vi "pco.camera_Live_ConvertSetting_Examples.vi"() -> ()   [LabVIEW 2019]
doc: "A short program to demonstrate the fundamentals of control and image acquision with the pco.camera series. The program records a sequence of images, with \"live\" updating, until the \"StopRecording\" button is pressed. Use ctrl-H for more help on the individual controls and indicators.\n\nCopyright 2004, 2010 The Cooke Corporation."
uses:
  pco.camera/Camera.lvclass
  pco.sdk/TimingControl/TimingControl.lvlib
  <vilib>/picture/picture.llb/Draw True-Color Pixmap.vi
  <vilib>/picture/picture.llb/Draw 8-Bit Pixmap.vi
panel:
  out "colormap(U8)":u32[](array[numeric])
  out "Image(U16)":u16[][](graph)
  in  "Zoom [%]":i32(c297)=26
  out "Image":picture
  in  "settingsChanged":bool
  in  "Trigger":bool
  in  "LUT File":path
  in  "data_format":T1(ring)=enum."RGBA8"
  in  "Auto Range":bool
  out "rawImage":u16[][](array[numeric])
  in  "iContrast [%]":i32 min=-100 max=99 step=1
  in  "Gamma":dbl=1.0 min=0.01 max=10.0 step=0.01 format="%.2f"
  in  "whiteBalance":bool
  in  "iScale_max":u16=60000 step=1
  in  "iScale_min":u16=200 step=1
  in  "Image Index":u32 max=9
  out "Recorded Images":u32
  in  "TriggerMode":T2(ring)
  in  "Quit":bool
  out "Error":errorcluster {"code" format="%x"}
  in  "Stop Record":bool
  out "Recording On":bool
  in  "roiY1":u64=2 min=1 max=2160 step=1
  in  "roiX1":u64=2 min=1 max=2560 step=1
  in  "roiY0":u64=1 min=1 max=2159 step=1
  in  "roiX0":u64=1 min=1 max=2559 step=1
  out "Image Height":u64
  out "Image Width":u64
  in  "dwImgCount":u32=10 caption="Required Number of Images" max=2397
  in  "Exposure Time [s]":dbl=0.010000000000000002 min=0.0005 max=2.0 step=0.001
  # "This example demonstrates the image acquisition with one camera in ring buffer mode together with a live display of the latest images during record. After record is stopped, the images can be addressed by index.\nAdditionally the image convert settings can be adjusted at any time\nNote that this example will not be fail save, i.e. doesnt react on errors, just handles them forward to the end\n\nUsage:\nSelect your required image count and the camera setup before you start the program.\nOnce started, the camera class will be initialized and images will be recorded and displayed automatically\nYou can stop the images by pressing stop record.\nAfter stopped, the image at the selected index will be read out\nTo finish the program click on quit application, this will force an exit of the camera class\nYou can change your required ROI after and also during the record."
  # "pco.labview"
  # "Camera Setup"
  # "Recording Control"
  # "Parameters for image readout"
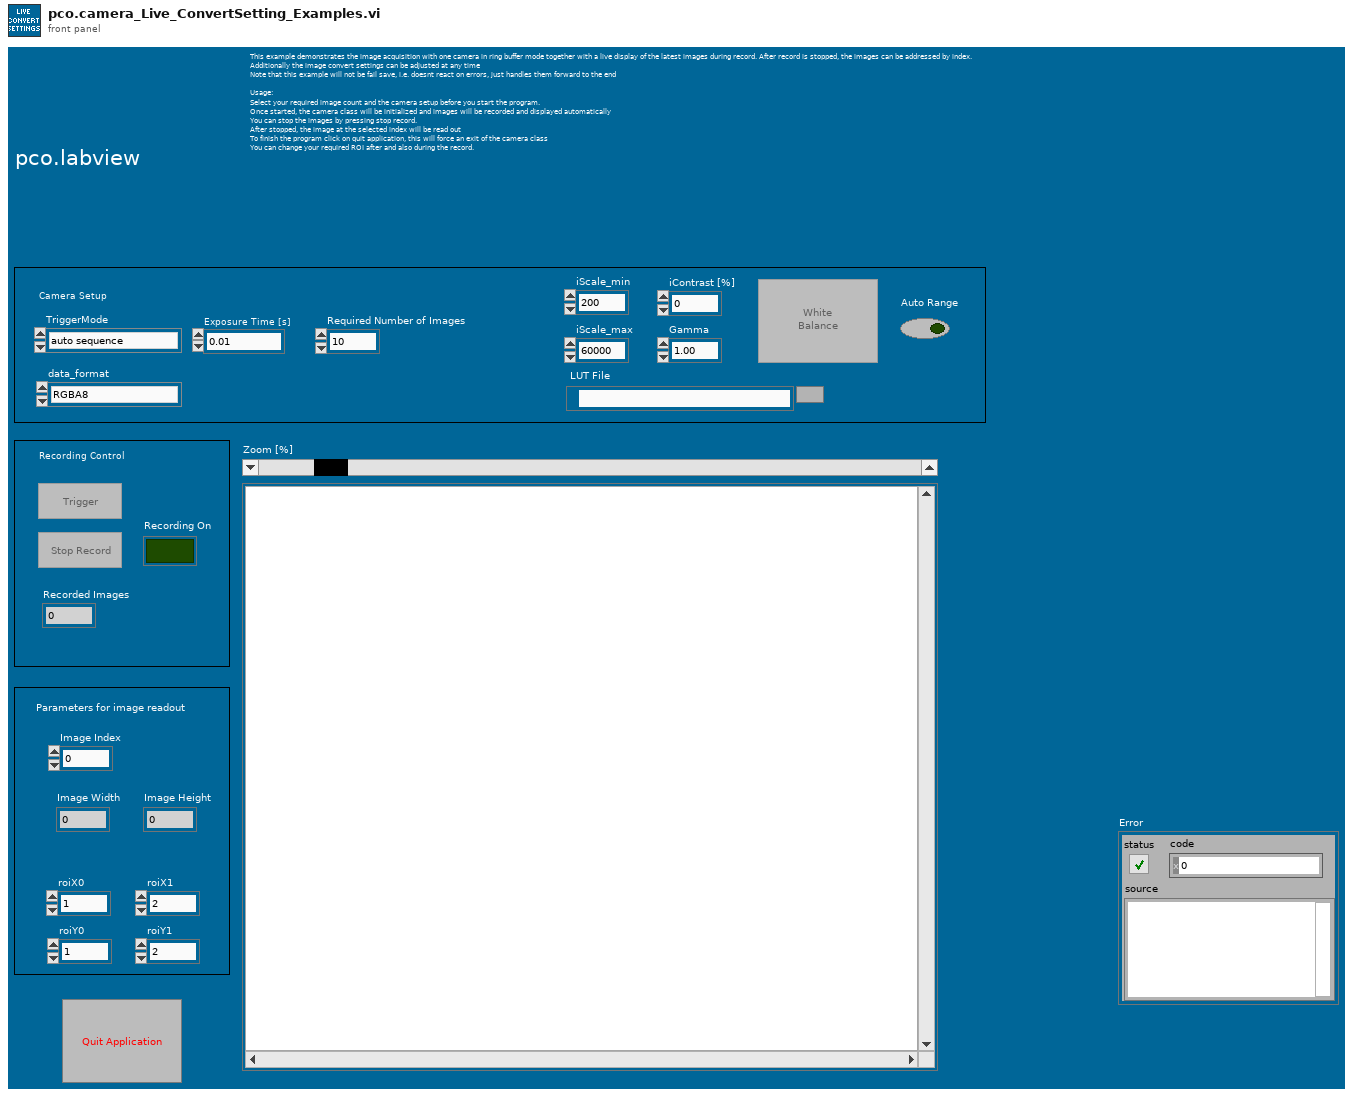
[diagram p1: front panel]
types:
  T1 = enum16{"Undefined", "Mono8", "Mono16", "BGRA8", "RGBA8", "BGRA16", "RGBA16", "CompressedMono8"}
  T2 = enum16{"auto sequence", "software trigger", "external exposure start", "external exposure control"}
  T3 = enum16{"sequence", "sequence non blocking", "ring buffer", "fifo", "sequence_dpcore", "sequence_non_blocking_dpcore", "ring_buffer_dpcore", "fifo_dpcore", "tif", "multitif", "pcoraw", "b16", "dicom", "multidicom"}
  T4 = enum8{"Enabled", "Disabled", "Disabled and Grayed Out"}
  T5 = cluster{"serial":u32, "type":u16, "sub_type":u16, "interface_type":u16, "bit_resolution":u16, "min_exposure_time_s":dbl, "max_exposure_time_s":dbl, "min_exposure_step_s":dbl, "min_delay_time_s":dbl, "max_delay_time_s":dbl, "min_delay_step_s":dbl, "min_width":u64, "min_height":u64, "max_width":u64, "max_height":u64, "roi_step_horz":u64, "roi_step_vert":u64, "roi_symmetric_horz":bool, "roi_symmetric_vert":bool, "has_timestamp_mode":bool, "has_timestamp_mode_ascii_only":bool, "pixelrate_vec":u32[], "has_acquire_mode":bool, "has_ext_acquire_mode":bool, "has_metadata_mode":bool, "has_ram":bool, "binning_horz_vec":u16[], "binning_vert_vec":u16[]}
  T6 = typedef "Camera.lvclass/binning.ctl" = cluster{"vert":u16, "horz":u16}
  T7 = cluster{"exposure_time_s":dbl, "delay_time_s":dbl, "roi":cluster{"x0":u64, "y0":u64, "x1":u64, "y1":u64}, "timestamp_mode":u16, "pixelrate":u32, "trigger_mode":u16, "acquire_mode":u16, "metadata_mode":u16, "noisefilter_mode":u16, "binning":T6}
  T8 = cluster{"sharpen":bool, "adaptive_sharpen":bool, "flip_vertical":bool, "auto_minmax":bool, "min_limit":u16, "max_limit":u16, "gamma":dbl, "contrast":i32, "pco_debayer_algorithm":bool, "color_temperature":i32, "color_saturation":i32, "color_vibrance":i32, "color_tint":i32, "lut_file":path}
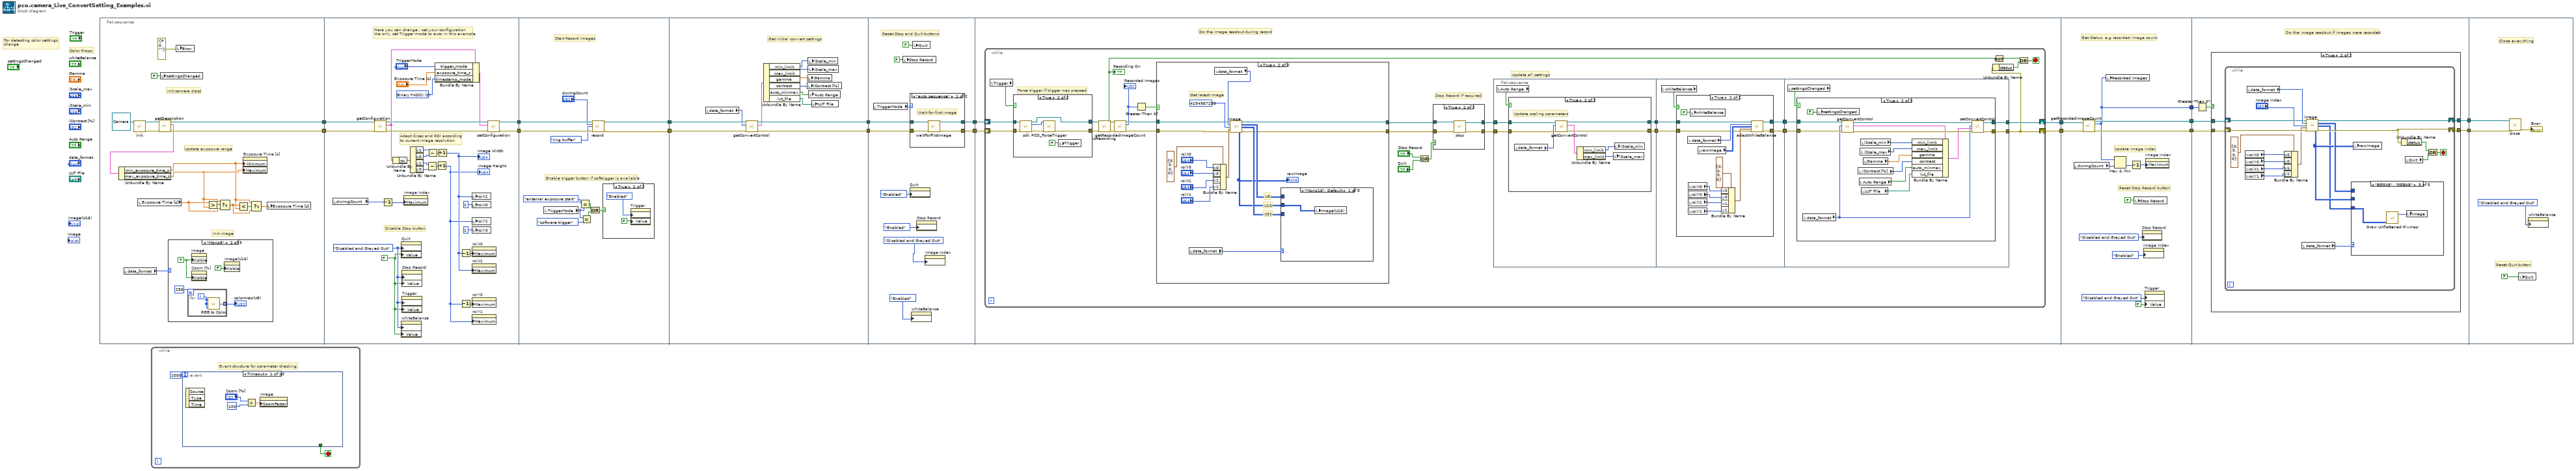
[diagram p0: block diagram]
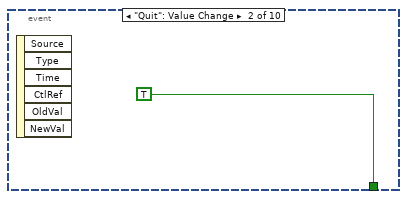
[diagram p2: hidden frame]
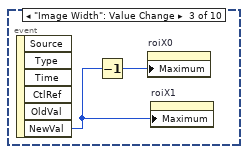
[diagram p3: hidden frame]
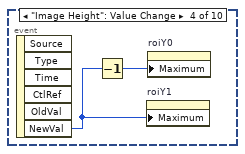
[diagram p4: hidden frame]
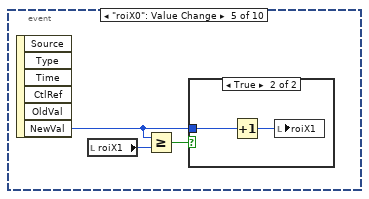
[diagram p5: hidden frame]
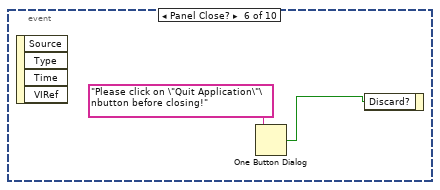
[diagram p7: hidden frame]
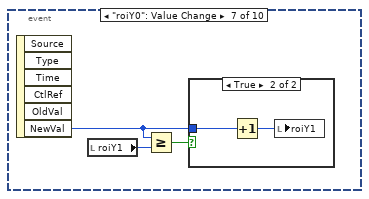
[diagram p8: hidden frame]
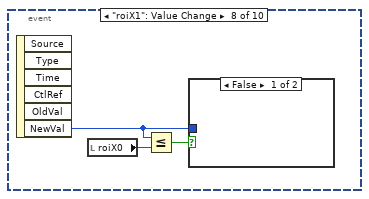
[diagram p10: hidden frame]
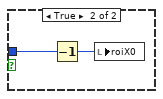
[diagram p11: hidden frame]
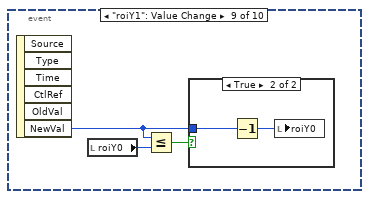
[diagram p12: hidden frame]
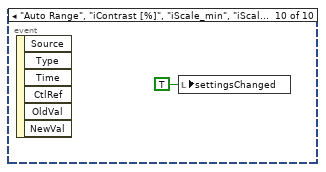
[diagram p14: hidden frame]
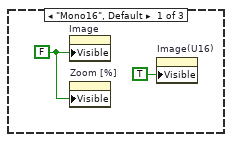
[diagram p15: hidden frame]
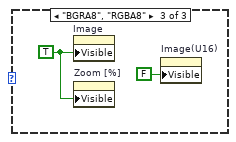
[diagram p16: hidden frame]
diagram:
  # "For detecting color settings\nchange"
  # "Color Props"
  n1 = flat-sequence {
    tunnel: [w24] -> w7
    tunnel: [w23] -> w6
    tunnel: [w48] -> w17
    tunnel: [w52] -> w16
    tunnel: w7 -> [w47]
    tunnel: w6 -> [w46]
    tunnel: w17 -> [w82]
    tunnel: w16 -> [w83]
    tunnel: [w79] -> w11
    tunnel: [w80] -> w8
    tunnel: w11 -> [w96]
    tunnel: [w91] -> w10
    tunnel: [w97] -> w9
    tunnel: w8 -> [w87]
    tunnel: w10 -> [w104]
    tunnel: w9 -> [w105]
    tunnel: [w103] -> w15
    tunnel: [w100] -> w2
    tunnel: w15 -> [w118]
    tunnel: [w117] -> w14
    tunnel: [w116] -> w5
    tunnel: w2 -> [w115]
    tunnel: w14 -> [w253]
    tunnel: [w251] -> w13
    tunnel: w5 -> [w246]
    tunnel: [w245] -> w4
    tunnel: [w244] -> w1
    tunnel: w13 -> [w262]
    tunnel: [w261] -> w12
    tunnel: w4 -> [w260]
    tunnel: [w259] -> w3
    tunnel: w1 -> [w257]
    tunnel: w12 -> [w297]
    tunnel: w3 -> [w294]
    frame #0 {
      # "Init image"
      # "Init camera class"
      # "Update exposure range"
      n2 = local read "data_format"() -> (w19:T1)
      n3 = call-dynamic "init.vi"("Camera in"=refnum<class "Camera.lvclass"> refnum) -> ("Camera out"=w25:refnum<class "Camera.lvclass">, "error out"=w26:errorcluster)  [unwired: 8 in]
      n4 = local read "Exposure Time [s]"() -> (w32:dbl)
      n5 = call-dynamic "getDescription.vi"("error in (no error)"=w26, "Camera in"=w25) -> ("error out"=w23:errorcluster, "description"=w22:T5, "Camera out"=w24:refnum<class "Camera.lvclass">)  [unwired: 7 in]
      n6 = Unbundle By Name(w22) -> ("min_exposure_time_s"=w21:dbl, "max_exposure_time_s"=w20:dbl)
      n7 = local write "settingsChanged"(FALSE ("settingsChanged")) -> ()
      n8 = case shown="\"Mono8\"" w19 {
        frame "Mono16", Default {
          w34 = FALSE ("Visible")
          n9 = property on="Image" class="Pict"("Visible"=w34) -> ()  [unwired: 2 in, 2 out]
          n10 = property on="Zoom [%]" class="Scroll (strict)"("Visible"=w34) -> ()  [unwired: 2 in, 2 out]
          n11 = property on="Image(U16)" class="IntGraph (strict)"("Visible"=TRUE) -> ()  [unwired: 2 in, 2 out]
        }
        frame "Mono8" {
          w36 = TRUE ("Visible")
          n12 = for {
            N: 256 -> [_]
            tunnel: [w40] -> w39 mode=indexing
            i -> [w41]
            n13 = call <vilib>:"RGB to Color.vi"("B"=w41, "G"=w41, "R"=w41) -> ("Color"=w40:u32)
          }
          "colormap(U8)" <- w39
          n14 = property on="Image" class="Pict"("Visible"=w36) -> ()  [unwired: 2 in, 2 out]
          n15 = property on="Zoom [%]" class="Scroll (strict)"("Visible"=w36) -> ()  [unwired: 2 in, 2 out]
          n16 = property on="Image(U16)" class="IntGraph (strict)"("Visible"=FALSE) -> ()  [unwired: 2 in, 2 out]
        }
        frame "BGRA8", "RGBA8" {
          w42 = TRUE ("Visible")
          n17 = property on="Image" class="Pict"("Visible"=w42) -> ()  [unwired: 2 in, 2 out]
          n18 = property on="Zoom [%]" class="Scroll (strict)"("Visible"=w42) -> ()  [unwired: 2 in, 2 out]
          n19 = property on="Image(U16)" class="IntGraph (strict)"("Visible"=FALSE) -> ()  [unwired: 2 in, 2 out]
        }
      }
      n20 = local write "Error"(errorcluster {"status"=FALSE, "code"=0, "source"=""} ("error IO")) -> ()
      n21 = Greater?(x=w32, y=w20) -> (0:w33:bool)
      n22 = Select(t=w20, s=w33, f=w32) -> (s? t:f=w30:dbl)
      n23 = Less?(x=w30, y=w21) -> (x < y?=w31:bool)
      n24 = property on="Exposure Time [s]" class="DigNum (strict)"("Minimum"=w21, "Maximum"=w20) -> ()  [unwired: 2 in, 2 out]
      n25 = Select(t=w21, s=w31, f=w30) -> (s? t:f=w29:dbl)
      n26 = local write "Exposure Time [s]"(w29) -> ()
    }
    frame #1 {
      w58 = u16 2 items=["OFF", "Binary", "Binary+ASCII", "ASCII"] ("wTimeStampMode")
      w44 = FALSE ("Stop")
      w45 = T4."Disabled and Grayed Out" ("Disabled")
      # "Disable Stop button"
      # "Adapt Sizes and ROI according\nto current image resolution"
      # "Here you can change / set your configuration\nWe only set Trigger mode to auto in this example"
      n27 = local read "dwImgCount"() -> (w59:u32)
      n28 = call-dynamic "getConfiguration.vi"("error in (no error)"=w46, "Camera in"=w47) -> ("error out"=w53:errorcluster, "configuration"=w64:T7, "Camera out"=w55:refnum<class "Camera.lvclass">)  [unwired: 7 in]
      n29 = Decrement(x=w59) -> (x-1=w49:u32)
      n30 = Unbundle By Name(w64) -> ("roi"=w65:cluster{"x0":u64, "y0":u64, "x1":u64, "y1":u64})
      n31 = property on="Quit" class="Bool (strict)"("DisabledEnum"=w45, "Value"=w44) -> ()  [unwired: 2 in, 2 out]
      n32 = property on="whiteBalance" class="Bool (strict)"("DisabledEnum"=w45, "Value"=w44) -> ()  [unwired: 2 in, 2 out]
      n33 = property on="Stop Record" class="Bool (strict)"("DisabledEnum"=w45, "Value"=w44) -> ()  [unwired: 2 in, 2 out]
      n34 = property on="Trigger" class="Bool (strict)"("DisabledEnum"=w45, "Value"=w44) -> ()  [unwired: 2 in, 2 out]
      n35 = property on="Image Index" class="DigNum (strict)"("Maximum"=w49) -> ()  [unwired: 2 in, 2 out]
      n36 = Unbundle By Name(w65) -> ("x1"=w67:u64, "x0"=w66:u64, "y1"=w69:u64, "y0"=w68:u64)
      n37 = Subtract(x=w69, y=w68) -> (x-y=w71:u64)
      n38 = Subtract(x=w67, y=w66) -> (x-y=w70:u64)
      n39 = Bundle By Name(cluster=w64, "trigger_mode"="TriggerMode", "exposure_time_s"="Exposure Time [s]", "timestamp_mode"=w58) -> (w54:T7)
      n40 = Increment(x=w71) -> (x+1=w50:u64)
      "Image Height" <- w50
      n41 = Increment(x=w70) -> (x+1=w51:u64)
      "Image Width" <- w51
      n42 = Decrement(x=w51) -> (x-1=w62:u64)
      n43 = Decrement(x=w50) -> (x-1=w63:u64)
      n44 = local write "roiX1"(w51) -> ()
      n45 = local write "roiX0"(u64 1 ("roiY0")) -> ()
      n46 = local write "roiY1"(w50) -> ()
      n47 = local write "roiY0"(u64 1 ("roiY0")) -> ()
      n48 = property on="roiX0" class="DigNum (strict)"("Maximum"=w62) -> ()  [unwired: 2 in, 2 out]
      n49 = property on="roiX1" class="DigNum (strict)"("Maximum"=w51) -> ()  [unwired: 2 in, 2 out]
      n50 = property on="roiY0" class="DigNum (strict)"("Maximum"=w63) -> ()  [unwired: 2 in, 2 out]
      n51 = property on="roiY1" class="DigNum (strict)"("Maximum"=w50) -> ()  [unwired: 2 in, 2 out]
      n52 = call-dynamic "setConfiguration.vi"("error in (no error)"=w53, "configuration"=w54, "Camera in"=w55) -> ("error out"=w52:errorcluster, "Camera out"=w48:refnum<class "Camera.lvclass">)  [unwired: 7 in]
    }
    frame #2 {
      # "Enable trigger button if softtrigger is available"
      # "Start Record Images"
      n53 = local read "TriggerMode"() -> (w77:T2)
      n54 = Equal?(x=T2."external exposure start" ("TriggerMode"), y=w77) -> (x = y?=w74:bool)
      n55 = Equal?(x=w77, y=T2."software trigger" ("TriggerMode")) -> (x = y?=w73:bool)
      n56 = Or(x=w74, y=w73) -> (x .or. y?=w75:bool)
      n57 = call-dynamic "record.vi"("Camera in"=w82, "num_images"="dwImgCount", "record_mode"=T3."ring buffer", "error in (no error)"=w83) -> ("Camera out"=w80:refnum<class "Camera.lvclass">, "error out"=w79:errorcluster)  [unwired: 10 in]
      n58 = case shown="True" w75 {
        frame False {
        }
        frame True {
          n59 = property on="Trigger" class="Bool (strict)"("DisabledEnum"=T4."Enabled" ("Disabled"), "Value"=FALSE ("Trigger")) -> ()  [unwired: 2 in, 2 out]
        }
      }
    }
    frame #3 {
      # "Get initial convert settings"
      n60 = local read "data_format"() -> (w86:T1)
      n61 = call-dynamic "getConvertControl.vi"("error in (no error)"=w96, "data_format"=w86, "Camera in"=w87) -> ("error out"=w91:errorcluster, "convert_control"=w95:T8, "Camera out"=w97:refnum<class "Camera.lvclass">)  [unwired: 6 in]
      n62 = Unbundle By Name(w95) -> ("min_limit"=w93:u16, "max_limit"=w92:u16, "gamma"=w94:dbl, "contrast"=w90:i32, "auto_minmax"=w89:bool, "lut_file"=w88:path)
      n63 = local write "iContrast [%]"(w90) -> ()
      n64 = local write "Gamma"(w94) -> ()
      n65 = local write "iScale_min"(w93) -> ()
      n66 = local write "iScale_max"(w92) -> ()
      n67 = local write "Auto Range"(w89) -> ()
      n68 = local write "LUT File"(w88) -> ()
    }
    frame #4 {
      # "Reset Stop and Quit buttons"
      n69 = local read "TriggerMode"() -> (w98:T2)
      n70 = local write "Stop Record"(FALSE ("Stop Record")) -> ()
      n71 = case shown="\"auto sequence\"" w98 {
        tunnel: w105 -> [w112 w114]
        tunnel: w104 -> [w111 w113]
        tunnel: [w110 w113] -> w103
        tunnel: [w109 w114] -> w100
        frame "auto sequence" {
          # "Wait for first image"
          n72 = call-dynamic "waitForFirstImage.vi"("error in (no error)"=w111, "Camera in"=w112) -> ("error out"=w110:errorcluster, "Camera out"=w109:refnum<class "Camera.lvclass">)  [unwired: 8 in]
        }
        frame Default {
          # "Don't wait \nif we trigger"
        }
      }
      n73 = property on="Quit" class="Bool (strict)"("DisabledEnum"=T4."Enabled" ("Disabled")) -> ()  [unwired: 2 in, 2 out]
      n74 = property on="whiteBalance" class="Bool (strict)"("DisabledEnum"=T4."Enabled" ("Disabled")) -> ()  [unwired: 2 in, 2 out]
      n75 = local write "Quit"(FALSE ("Stop")) -> ()
      n76 = property on="Stop Record" class="Bool (strict)"("DisabledEnum"=T4."Enabled" ("Disabled")) -> ()  [unwired: 2 in, 2 out]
      n77 = property on="Image Index" class="DigNum (strict)"("DisabledEnum"=T4."Disabled and Grayed Out" ("Disabled")) -> ()  [unwired: 2 in, 2 out]
    }
    frame #5 {
      # "Do the image readout during record"
      n78 = while {
        shift-right: [w128] -> w117
        shift-left: w118 -> [w131]
        shift-right: [w134] -> w116
        shift-left: w115 -> [w132]
        stop <- w146 stop-if-true
        # "Stop Record if required"
        # "Force trigger if trigger was pressed"
        # "Update all settings"
        n79 = local read "Trigger"() -> (w133:bool)
        n80 = case shown="True" w133 {
          tunnel: w132 -> [w178 w183]
          tunnel: w131 -> [w177 w182]
          tunnel: [w178 w181] -> w130
          tunnel: [w177 w180] -> w129
          frame False {
          }
          frame True {
            n81 = call-dynamic "sdk.vi"("Camera in"=w183, "error in (no error)"=w182) -> ("Camera out"=w181:refnum<class "Camera.lvclass">, "sdk"=w184:u64, "error out"=w185:errorcluster)  [unwired: 11 in]
            n82 = call "PCO_ForceTrigger.vi"("error in (no error)"=w185, "ph"=w184) -> ("error out"=w180:errorcluster)  [unwired: 6 in, 3 out]
            n83 = local write "Trigger"(FALSE ("Trigger")) -> ()
          }
        }
        n84 = call-dynamic "isRecording.vi"("Camera in"=w130, "error in (no error)"=w129) -> ("Camera out"=w142:refnum<class "Camera.lvclass">, "recording"=w144:bool, "error out"=w141:errorcluster)  [unwired: 11 in]
        "Recording On" <- w144
        n85 = call-dynamic "getRecordedImageCount.vi"("Camera in"=w142, "error in (no error)"=w141) -> ("Camera out"=w139:refnum<class "Camera.lvclass">, "recorded_image_count"=w127:u32, "error out"=w140:errorcluster)  [unwired: 11 in]
        "Recorded Images" <- w127
        n86 = Greater Than 0?(x=w127) -> (x > 0?=w126:bool)
        n87 = case shown="True" w126 {
          tunnel: w140 -> [w153 w163]
          tunnel: w139 -> [w154 w157]
          tunnel: [w153 w155] -> w122
          tunnel: [w154 w156] -> w121
          frame False {
          }
          frame True {
            # "U32"
            # "U8"
            # "U16"
            # "Get latest image"
            n88 = local read "data_format"() -> (w158:T1)
            n89 = Bundle By Name(cluster=cluster{"x0":u64, "y0":u64, "x1":u64, "y1":u64} {"x0"=0, "y0"=0, "x1"=0, "y1"=0} ("roi"), "x0"="roiX0", "y0"="roiY0", "x1"="roiX1", "y1"="roiY1") -> (w166:cluster{"x0":u64, "y0":u64, "x1":u64, "y1":u64})
            n90 = local read "data_format"() -> (w162:T1)
            n91 = call-dynamic "image.vi"("Camera in"=w157, "data_format"=w162, "image_index"=u32 4294967295 ("dwImgIdx"), "roi"=w166, "error in (no error)"=w163) -> ("Camera out"=w156:refnum<class "Camera.lvclass">, "image (U8)"=w160:u8[][], "image (U32)"=w161:u32[][], "raw_image (U16)"=w159:u16[][], "error out"=w155:errorcluster)  [unwired: 3 in, 3 out]
            "rawImage" <- w159
            n92 = case shown="\"Mono16\", Default" w158 {
              tunnel: w161 -> [_ _ w176]
              tunnel: w160 -> [_ w173 _]
              tunnel: w159 -> [w171 _ _]
              frame "Mono16", Default {
                n93 = local write "Image(U16)"(w171) -> ()
              }
              frame "Mono8" {
                n94 = local read "colormap(U8)"() -> (w172:u32[])
                n95 = call-poly <vilib>:"Draw Unflattened Pixmap.vi"("data"=w173, "color table"=w172) -> ("new picture"=w174:picture)  [unwired: 7 in]
                n96 = local write "Image"(w174) -> ()
              }
              frame "BGRA8", "RGBA8" {
                n97 = call-poly <vilib>:"Draw Unflattened Pixmap.vi"("data (RGB format)"=w176) -> ("new picture"=w175:picture)  [unwired: 8 in]
                n98 = local write "Image"(w175) -> ()
              }
            }
          }
        }
        n99 = Or(x="Stop Record", y="Quit") -> (x .or. y?=w125:bool)
        n100 = case shown="True" w125 {
          tunnel: w122 -> [w148 w149]
          tunnel: [w147 w151] -> w120
          tunnel: [w148 w152] -> w119
          tunnel: w121 -> [w147 w150]
          frame False {
          }
          frame True {
            n101 = call-dynamic "stop.vi"("error in (no error)"=w149, "Camera in"=w150) -> ("error out"=w152:errorcluster, "Camera out"=w151:refnum<class "Camera.lvclass">)  [unwired: 8 in]
          }
        }
        n102 = flat-sequence {
          tunnel: w119 -> [w188]
          tunnel: w120 -> [w189]
          tunnel: [w187] -> w138
          tunnel: [w186] -> w137
          tunnel: w138 -> [w204]
          tunnel: w137 -> [w203]
          tunnel: [w202] -> w136
          tunnel: [w201] -> w135
          tunnel: w136 -> [w223]
          tunnel: w135 -> [w224]
          tunnel: [w222] -> w128
          tunnel: [w221] -> w134
          frame #0 {
            n103 = local read "Auto Range"() -> (w190:bool)
            n104 = case shown="True" w190 {
              tunnel: w189 -> [w192 w196]
              tunnel: w188 -> [w191 w195]
              tunnel: [w191 w194] -> w187
              tunnel: [w192 w193] -> w186
              frame False {
              }
              frame True {
                # "Update scaling parameters"
                n105 = local read "data_format"() -> (w200:T1)
                n106 = call-dynamic "getConvertControl.vi"("error in (no error)"=w195, "data_format"=w200, "Camera in"=w196) -> ("error out"=w194:errorcluster, "convert_control"=w197:T8, "Camera out"=w193:refnum<class "Camera.lvclass">)  [unwired: 6 in]
                n107 = Unbundle By Name(w197) -> ("min_limit"=w198:u16, "max_limit"=w199:u16)
                n108 = local write "iScale_max"(w199) -> ()
                n109 = local write "iScale_min"(w198) -> ()
              }
            }
          }
          frame #1 {
            n110 = local read "whiteBalance"() -> (w205:bool)
            n111 = case shown="True" w205 {
              tunnel: w204 -> [w206 w212]
              tunnel: w203 -> [w207 w211]
              tunnel: [w206 w210] -> w202
              tunnel: [w207 w209] -> w201
              frame False {
              }
              frame True {
                n112 = local read "data_format"() -> (w219:T1)
                n113 = local read "roiX0"() -> (w217:u64)
                n114 = local read "roiY0"() -> (w216:u64)
                n115 = local read "roiX1"() -> (w215:u64)
                n116 = local read "roiY1"() -> (w208:u64)
                n117 = local write "whiteBalance"(FALSE ("whiteBalance")) -> ()
                n118 = local read "rawImage"() -> (w218:u16[][])
                n119 = Bundle By Name(cluster=cluster{"x0":u64, "y0":u64, "x1":u64, "y1":u64} {"x0"=0, "y0"=0, "x1"=0, "y1"=0} ("roi"), "x0"=w217, "y0"=w216, "x1"=w215, "y1"=w208) -> (w214:cluster{"x0":u64, "y0":u64, "x1":u64, "y1":u64})
                n120 = call-dynamic "adaptWhiteBalance.vi"("Camera in"=w211, "data_format"=w219, "raw_image (U16)"=w218, "roi"=w214, "error in (no error)"=w212) -> ("Camera out"=w209:refnum<class "Camera.lvclass">, "error out"=w210:errorcluster)  [unwired: 9 in]
              }
            }
          }
          frame #2 {
            n121 = local read "settingsChanged"() -> (w225:bool)
            n122 = case shown="True" w225 {
              tunnel: w224 -> [w227 w233]
              tunnel: w223 -> [w226 w232]
              tunnel: [w226 w229] -> w222
              tunnel: [w227 w228] -> w221
              frame False {
              }
              frame True {
                n123 = local read "data_format"() -> (w231:T1)
                n124 = local write "settingsChanged"(FALSE ("whiteBalance")) -> ()
                n125 = call-dynamic "getConvertControl.vi"("error in (no error)"=w232, "data_format"=w231, "Camera in"=w233) -> ("error out"=w235:errorcluster, "convert_control"=w242:T8, "Camera out"=w236:refnum<class "Camera.lvclass">)  [unwired: 6 in]
                n126 = local read "iContrast [%]"() -> (w238:i32)
                n127 = local read "Auto Range"() -> (w237:bool)
                n128 = local read "iScale_max"() -> (w240:u16)
                n129 = local read "iScale_min"() -> (w241:u16)
                n130 = local read "LUT File"() -> (w230:path)
                n131 = local read "Gamma"() -> (w239:dbl)
                n132 = Bundle By Name(cluster=w242, "min_limit"=w241, "max_limit"=w240, "gamma"=w239, "contrast"=w238, "auto_minmax"=w237, "lut_file"=w230) -> (w234:T8)
                n133 = call-dynamic "setConvertControl.vi"("error in (no error)"=w235, "convert_control"=w234, "data_format"=w231, "Camera in"=w236) -> ("error out"=w229:errorcluster, "Camera out"=w228:refnum<class "Camera.lvclass">)  [unwired: 6 in]
              }
            }
          }
        }
        n134 = Unbundle By Name(w128) -> ("status"=w145:bool)
        n135 = Not(x=w144) -> (.not. x?=w143:bool)
        n136 = Or(x=w143, y=w145) -> (x .or. y?=w146:bool)
      }
    }
    frame #6 {
      # "Update image index"
      # "Reset Stop Record button"
      # "Get Status, e.g recorded image count"
      n137 = local read "dwImgCount"() -> (w252:u32)
      n138 = call-dynamic "getRecordedImageCount.vi"("Camera in"=w246, "error in (no error)"=w253) -> ("Camera out"=w245:refnum<class "Camera.lvclass">, "recorded_image_count"=w244:u32, "error out"=w251:errorcluster)  [unwired: 11 in]
      n139 = local write "Recorded Images"(w244) -> ()
      n140 = Max & Min(x=w244, y=w252) -> (min(x,y)=w254:u32)  [unwired: 1 out]
      n141 = Decrement(x=w254) -> (x-1=w249:u32)
      n142 = local write "Stop Record"(FALSE ("Stop Record")) -> ()
      n143 = property on="Stop Record" class="Bool (strict)"("DisabledEnum"=T4."Disabled and Grayed Out" ("Disabled")) -> ()  [unwired: 2 in, 2 out]
      n144 = property on="Image Index" class="DigNum (strict)"("DisabledEnum"=T4."Enabled" ("Disabled")) -> ()  [unwired: 2 in, 2 out]
      n145 = property on="Trigger" class="Bool (strict)"("DisabledEnum"=T4."Disabled and Grayed Out" ("Disabled"), "Value"=FALSE ("Trigger")) -> ()  [unwired: 2 in, 2 out]
      n146 = property on="Image Index" class="DigNum (strict)"("Maximum"=w249) -> ()  [unwired: 2 in, 2 out]
    }
    frame #7 {
      # "Do the image readout if images were recorded"
      n147 = Greater Than 0?(x=w257) -> (x > 0?=w258:bool)
      n148 = case shown="True" w258 {
        tunnel: w262 -> [w263 w268]
        tunnel: [w263 w267] -> w261
        tunnel: w260 -> [w264 w266]
        tunnel: [w264 w265] -> w259
        frame False {
        }
        frame True {
          n149 = while {
            shift-right: [w279] -> w267
            shift-left: w268 -> [w287]
            shift-right: [w273] -> w265
            shift-left: w266 -> [w274]
            stop <- w281 stop-if-true
            n150 = local read "roiX0"() -> (w277:u64)
            n151 = local read "roiY0"() -> (w278:u64)
            n152 = local read "roiX1"() -> (w285:u64)
            n153 = local read "roiY1"() -> (w284:u64)
            n154 = local read "data_format"() -> (w275:T1)
            n155 = Bundle By Name(cluster=cluster{"x0":u64, "y0":u64, "x1":u64, "y1":u64} {"x0"=0, "y0"=0, "x1"=0, "y1"=0} ("roi"), "x0"=w277, "y0"=w278, "x1"=w285, "y1"=w284) -> (w286:cluster{"x0":u64, "y0":u64, "x1":u64, "y1":u64})
            n156 = local read "data_format"() -> (w269:T1)
            n157 = call-dynamic "image.vi"("Camera in"=w274, "data_format"=w275, "image_index"="Image Index", "roi"=w286, "error in (no error)"=w287) -> ("Camera out"=w273:refnum<class "Camera.lvclass">, "image (U8)"=w272:u8[][], "image (U32)"=w270:u32[][], "raw_image (U16)"=w271:u16[][], "error out"=w279:errorcluster)  [unwired: 3 in, 3 out]
            n158 = case shown="\"BGRA8\", \"RGBA8\"" w269 {
              tunnel: w270 -> [_ _ w293]
              tunnel: w272 -> [_ w290 _]
              tunnel: w271 -> [w288 _ _]
              frame "Mono16", Default {
                n159 = local write "Image(U16)"(w288) -> ()
              }
              frame "Mono8" {
                n160 = local read "colormap(U8)"() -> (w289:u32[])
                n161 = call-poly <vilib>:"Draw Unflattened Pixmap.vi"("data"=w290, "color table"=w289) -> ("new picture"=w291:picture)  [unwired: 7 in]
                n162 = local write "Image"(w291) -> ()
              }
              frame "BGRA8", "RGBA8" {
                n163 = call-poly <vilib>:"Draw Unflattened Pixmap.vi"("data (RGB format)"=w293) -> ("new picture"=w292:picture)  [unwired: 8 in]
                n164 = local write "Image"(w292) -> ()
              }
            }
            n165 = local write "rawImage"(w271) -> ()
            n166 = Unbundle By Name(w279) -> ("status"=w282:bool)
            n167 = local read "Quit"() -> (w283:bool)
            n168 = Or(x=w282, y=w283) -> (x .or. y?=w281:bool)
          }
        }
      }
    }
    frame #8 {
      # "Close everything"
      # "Reset Quit button"
      n169 = call-dynamic "close.vi"("error in (no error)"=w297, "Camera in"=w294) -> ("error out"=→"Error":errorcluster)  [unwired: 9 in]
      n170 = local write "Quit"(FALSE ("Stop Record")) -> ()
      n171 = property on="whiteBalance" class="Bool (strict)"("DisabledEnum"=T4."Disabled and Grayed Out" ("Disabled")) -> ()  [unwired: 2 in, 2 out]
    }
  }
  n172 = while {
    stop <- w299 stop-if-true
    # "Event structure for parameter checking"
    n173 = event shown="[0] Timeout" {
      selector: _ -> [_ _ _ _ _ _ _ _ _ _]
      dyn-events: _ -> [_ _ _ _ _ _ _ _ _ _]
      timeout: 1000 -> [_ _ _ _ _ _ _ _ _ _]
      tunnel: [_ TRUE _ _ _ _ _ _ _ _] -> w299
      event Timeout {
        n174 = event-data() -> ()  [unwired: 1 in, 3 out]
        n175 = Divide(x="Zoom [%]", y=100 ("Zoom [%]")) -> (x/y=w303:dbl)
        n176 = property on="Image" class="Pict"("ZoomFactor"=w303) -> ()  [unwired: 2 in, 2 out]
      }
      event "Quit": Value Change {
        n177 = event-data() -> ()  [unwired: 1 in, 6 out]
      }
      event "Image Width": Value Change {
        n178 = event-data() -> ("NewVal"=w305:u64)  [unwired: 1 in, 5 out]
        n179 = Decrement(x=w305) -> (x-1=w306:u64)
        n180 = property on="roiX0" class="DigNum (strict)"("Maximum"=w306) -> ()  [unwired: 2 in, 2 out]
        n181 = property on="roiX1" class="DigNum (strict)"("Maximum"=w305) -> ()  [unwired: 2 in, 2 out]
      }
      event "Image Height": Value Change {
        n182 = event-data() -> ("NewVal"=w307:u64)  [unwired: 1 in, 5 out]
        n183 = Decrement(x=w307) -> (x-1=w308:u64)
        n184 = property on="roiY1" class="DigNum (strict)"("Maximum"=w307) -> ()  [unwired: 2 in, 2 out]
        n185 = property on="roiY0" class="DigNum (strict)"("Maximum"=w308) -> ()  [unwired: 2 in, 2 out]
      }
      event "roiX0": Value Change {
        n186 = event-data() -> ("NewVal"=w309:u64)  [unwired: 1 in, 5 out]
        n187 = local read "roiX1"() -> (w311:u64)
        n188 = Greater Or Equal?(x=w309, y=w311) -> (x >= y?=w310:bool)
        n189 = case shown="True" w310 {
          tunnel: w309 -> [_ w313]
          frame False {
          }
          frame True {
            n190 = Increment(x=w313) -> (x+1=w312:u64)
            n191 = local write "roiX1"(w312) -> ()
          }
        }
      }
      event Panel Close? {
        n192 = event-data() -> ()  [unwired: 1 in, 4 out]
        n193 = One Button Dialog(message="Please click on \"Quit Application\"\nbutton before closing!") -> (true=w314:bool)  [unwired: 1 in]
        n194 = event-data("Discard?"=w314) -> ()  [unwired: 1 in, 1 out]
      }
      event "roiY0": Value Change {
        n195 = event-data() -> ("NewVal"=w316:u64)  [unwired: 1 in, 5 out]
        n196 = local read "roiY1"() -> (w318:u64)
        n197 = Greater Or Equal?(x=w316, y=w318) -> (x >= y?=w317:bool)
        n198 = case shown="True" w317 {
          tunnel: w316 -> [_ w320]
          frame False {
          }
          frame True {
            n199 = Increment(x=w320) -> (x+1=w319:u64)
            n200 = local write "roiY1"(w319) -> ()
          }
        }
      }
      event "roiX1": Value Change {
        n201 = event-data() -> ("NewVal"=w321:u64)  [unwired: 1 in, 5 out]
        n202 = local read "roiX0"() -> (w323:u64)
        n203 = Less Or Equal?(x=w321, y=w323) -> (x <= y?=w322:bool)
        n204 = case shown="False" w322 {
          tunnel: w321 -> [_ w325]
          frame False {
          }
          frame True {
            n205 = Decrement(x=w325) -> (x-1=w324:u64)
            n206 = local write "roiX0"(w324) -> ()
          }
        }
      }
      event "roiY1": Value Change {
        n207 = event-data() -> ("NewVal"=w326:u64)  [unwired: 1 in, 5 out]
        n208 = local read "roiY0"() -> (w328:u64)
        n209 = Less Or Equal?(x=w326, y=w328) -> (x <= y?=w327:bool)
        n210 = case shown="True" w327 {
          tunnel: w326 -> [_ w330]
          frame False {
          }
          frame True {
            n211 = Decrement(x=w330) -> (x-1=w329:u64)
            n212 = local write "roiY0"(w329) -> ()
          }
        }
      }
      event "Auto Range", "iContrast [%]", "iScale_min", "iScale_max", "Gamma", "LUT File": Value Change {
        n213 = event-data() -> ()  [unwired: 1 in, 6 out]
        n214 = local write "settingsChanged"(TRUE ("settingsChanged")) -> ()
      }
    }
  }
